vi "UI.vi"() -> ()   [LabVIEW 2016, in "动力环境.lvlib"]
uses:
  C:/Program Files (x86)/National Instruments/LabVIEW 2016/vi.lib/ActorFramework/Actor/Actor.lvclass
  DAM0200-Relay/DAM0200-Relay/DAM0200-Relay.lvclass
  EPEVER-MPPT/EPEVER-MPPT/EPEVER-MPPT.lvclass
  GPS/GPS/GPS.lvclass
  GPS/GPS/GPS.lvclass/GPS.ctl
  EPEVER-MPPT/EPEVER-MPPT/EPEVER-MPPT.lvclass/EPEVER-MPPT.ctl
  DAM0200-Relay/DAM0200-Relay/DAM0200-Relay.lvclass/DAM0200-Relay.ctl
  <vilib>/ActorFramework/Message Enqueuer/Message Enqueuer.lvclass/Message Enqueuer.ctl
  <vilib>/ActorFramework/Message Enqueuer/Enqueue.vi
  C:/Program Files (x86)/National Instruments/LabVIEW 2016/vi.lib/ActorFramework/Message/Message.lvclass
  <vilib>/ActorFramework/Stop Msg/Stop Msg.lvclass
  <vilib>/ActorFramework/Message Priority Queue/Priority Enqueue.vi
  <vilib>/ActorFramework/Actor/Actor.lvclass
  <vilib>/ptbypt/NI_PtbyPt.lvlib
  <vilib>/Utility/config.llb/NI_LVConfig.lvlib
panel:
  in  "仪器自动断电":T1={"开关"=enum."关闭", "偏置"=0, "间隔"=30} {"间隔" format="%02.0f"; "偏置" format="%02.0f"}
  out "通电时间":dbl format="%#.1f"
  out "偏移距离":dbl
  out "起始GPS":cluster{"GPS纬度":dbl[], "GPS经度":dbl[]} {"GPS经度" format="%#.6f °"; "GPS纬度" format="%#.6f °"}
  out "GPS轨迹图":cluster{"GPS纬度":dbl[], "GPS经度":dbl[]}[](graph)
  in  "仪器电源开关":bool
  in  "摄像头电源开关":bool
  out "仪器电源":bool
  out "摄像头电源":bool
  in  "GPS纬度":dbl format="%#.6f °"
  in  "GPS经度":dbl format="%#.6f °"
  in  "电压":dbl format="%#.2f V"
  in  "湿度":dbl format="%#.2f %%"
  in  "温度":dbl format="%#.2f ℃"
  # "开关："
  # "起始（分）："
  # "间隔（分）："
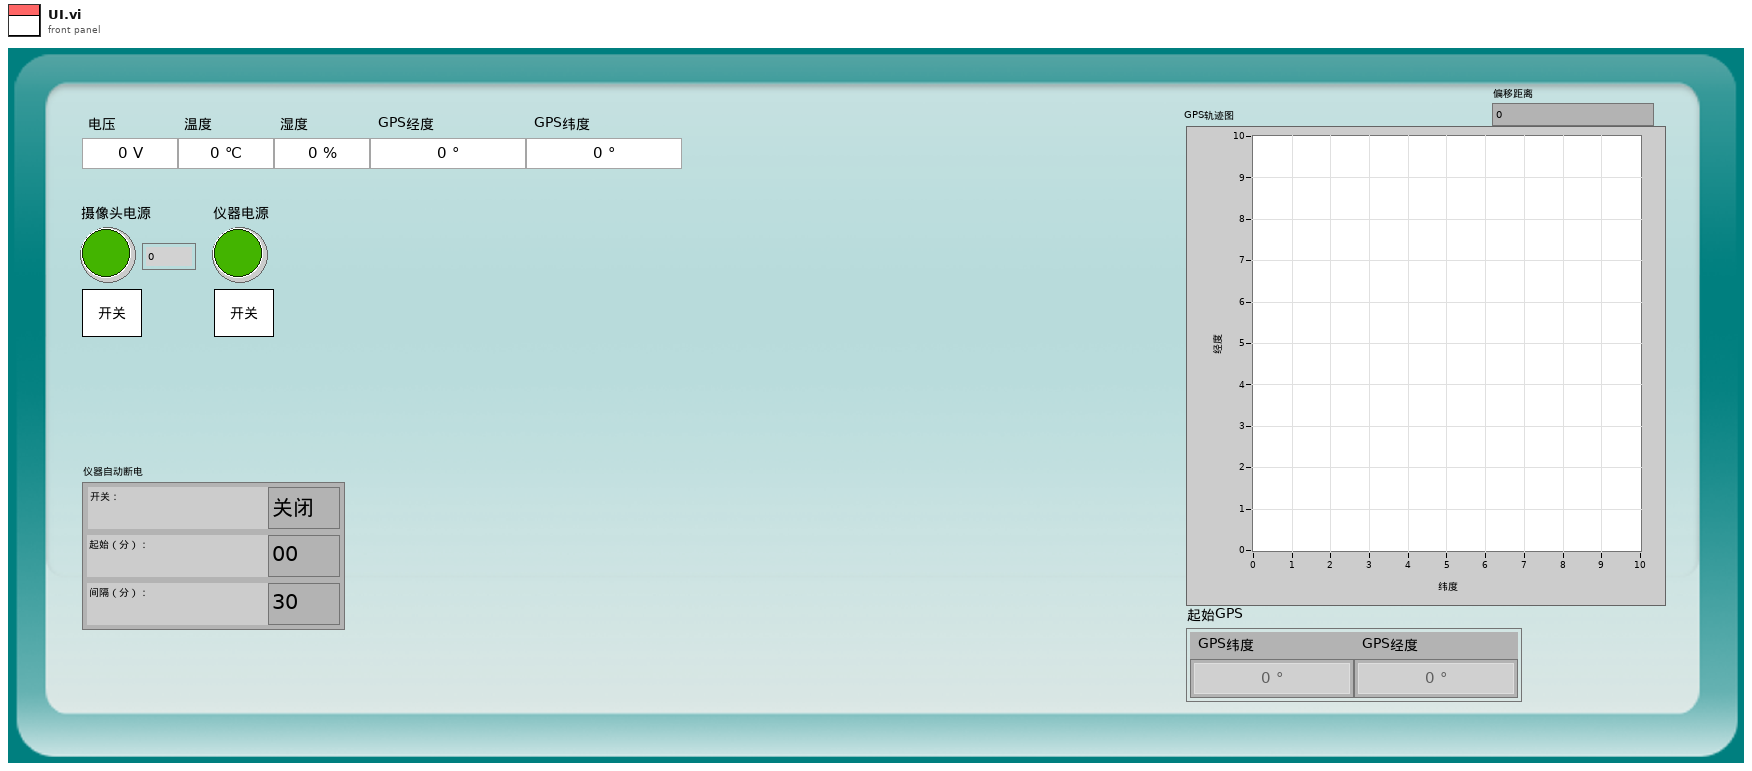
[diagram p1: front panel]
types:
  T1 = cluster{"开关":enum16{"关闭", "打开"}, "偏置":u16, "间隔":u16}
  T2 = cluster{"通电时间":timestamp, "通电超时？":bool, "低电压？":bool}
  T3 = typedef "报警信息字段定义.ctl" = cluster{"时间":timestamp, "参数":string, "元器件":string, "故障现象":string, "故障分析":string, "state":string, "code":string, "platform_alarm_code":string}
  T4 = typedef "NI_LVConfig.lvlib/Config Data RefNum.ctl" = refnum<k1>
  T5 = cluster{"时间":timestamp, "电压":dbl, "室温":dbl, "湿度":dbl, "GPS经度":dbl, "GPS纬度":dbl}
  T6 = typedef "LVDateTimeRec.ctl" = cluster{"秒数的小数部分":dbl, "秒":i32, "分":i32, "时":i32, "日":i32, "月":i32, "年":i32, "天数（周）":i32, "天数（年）":i32, "DST":i32}
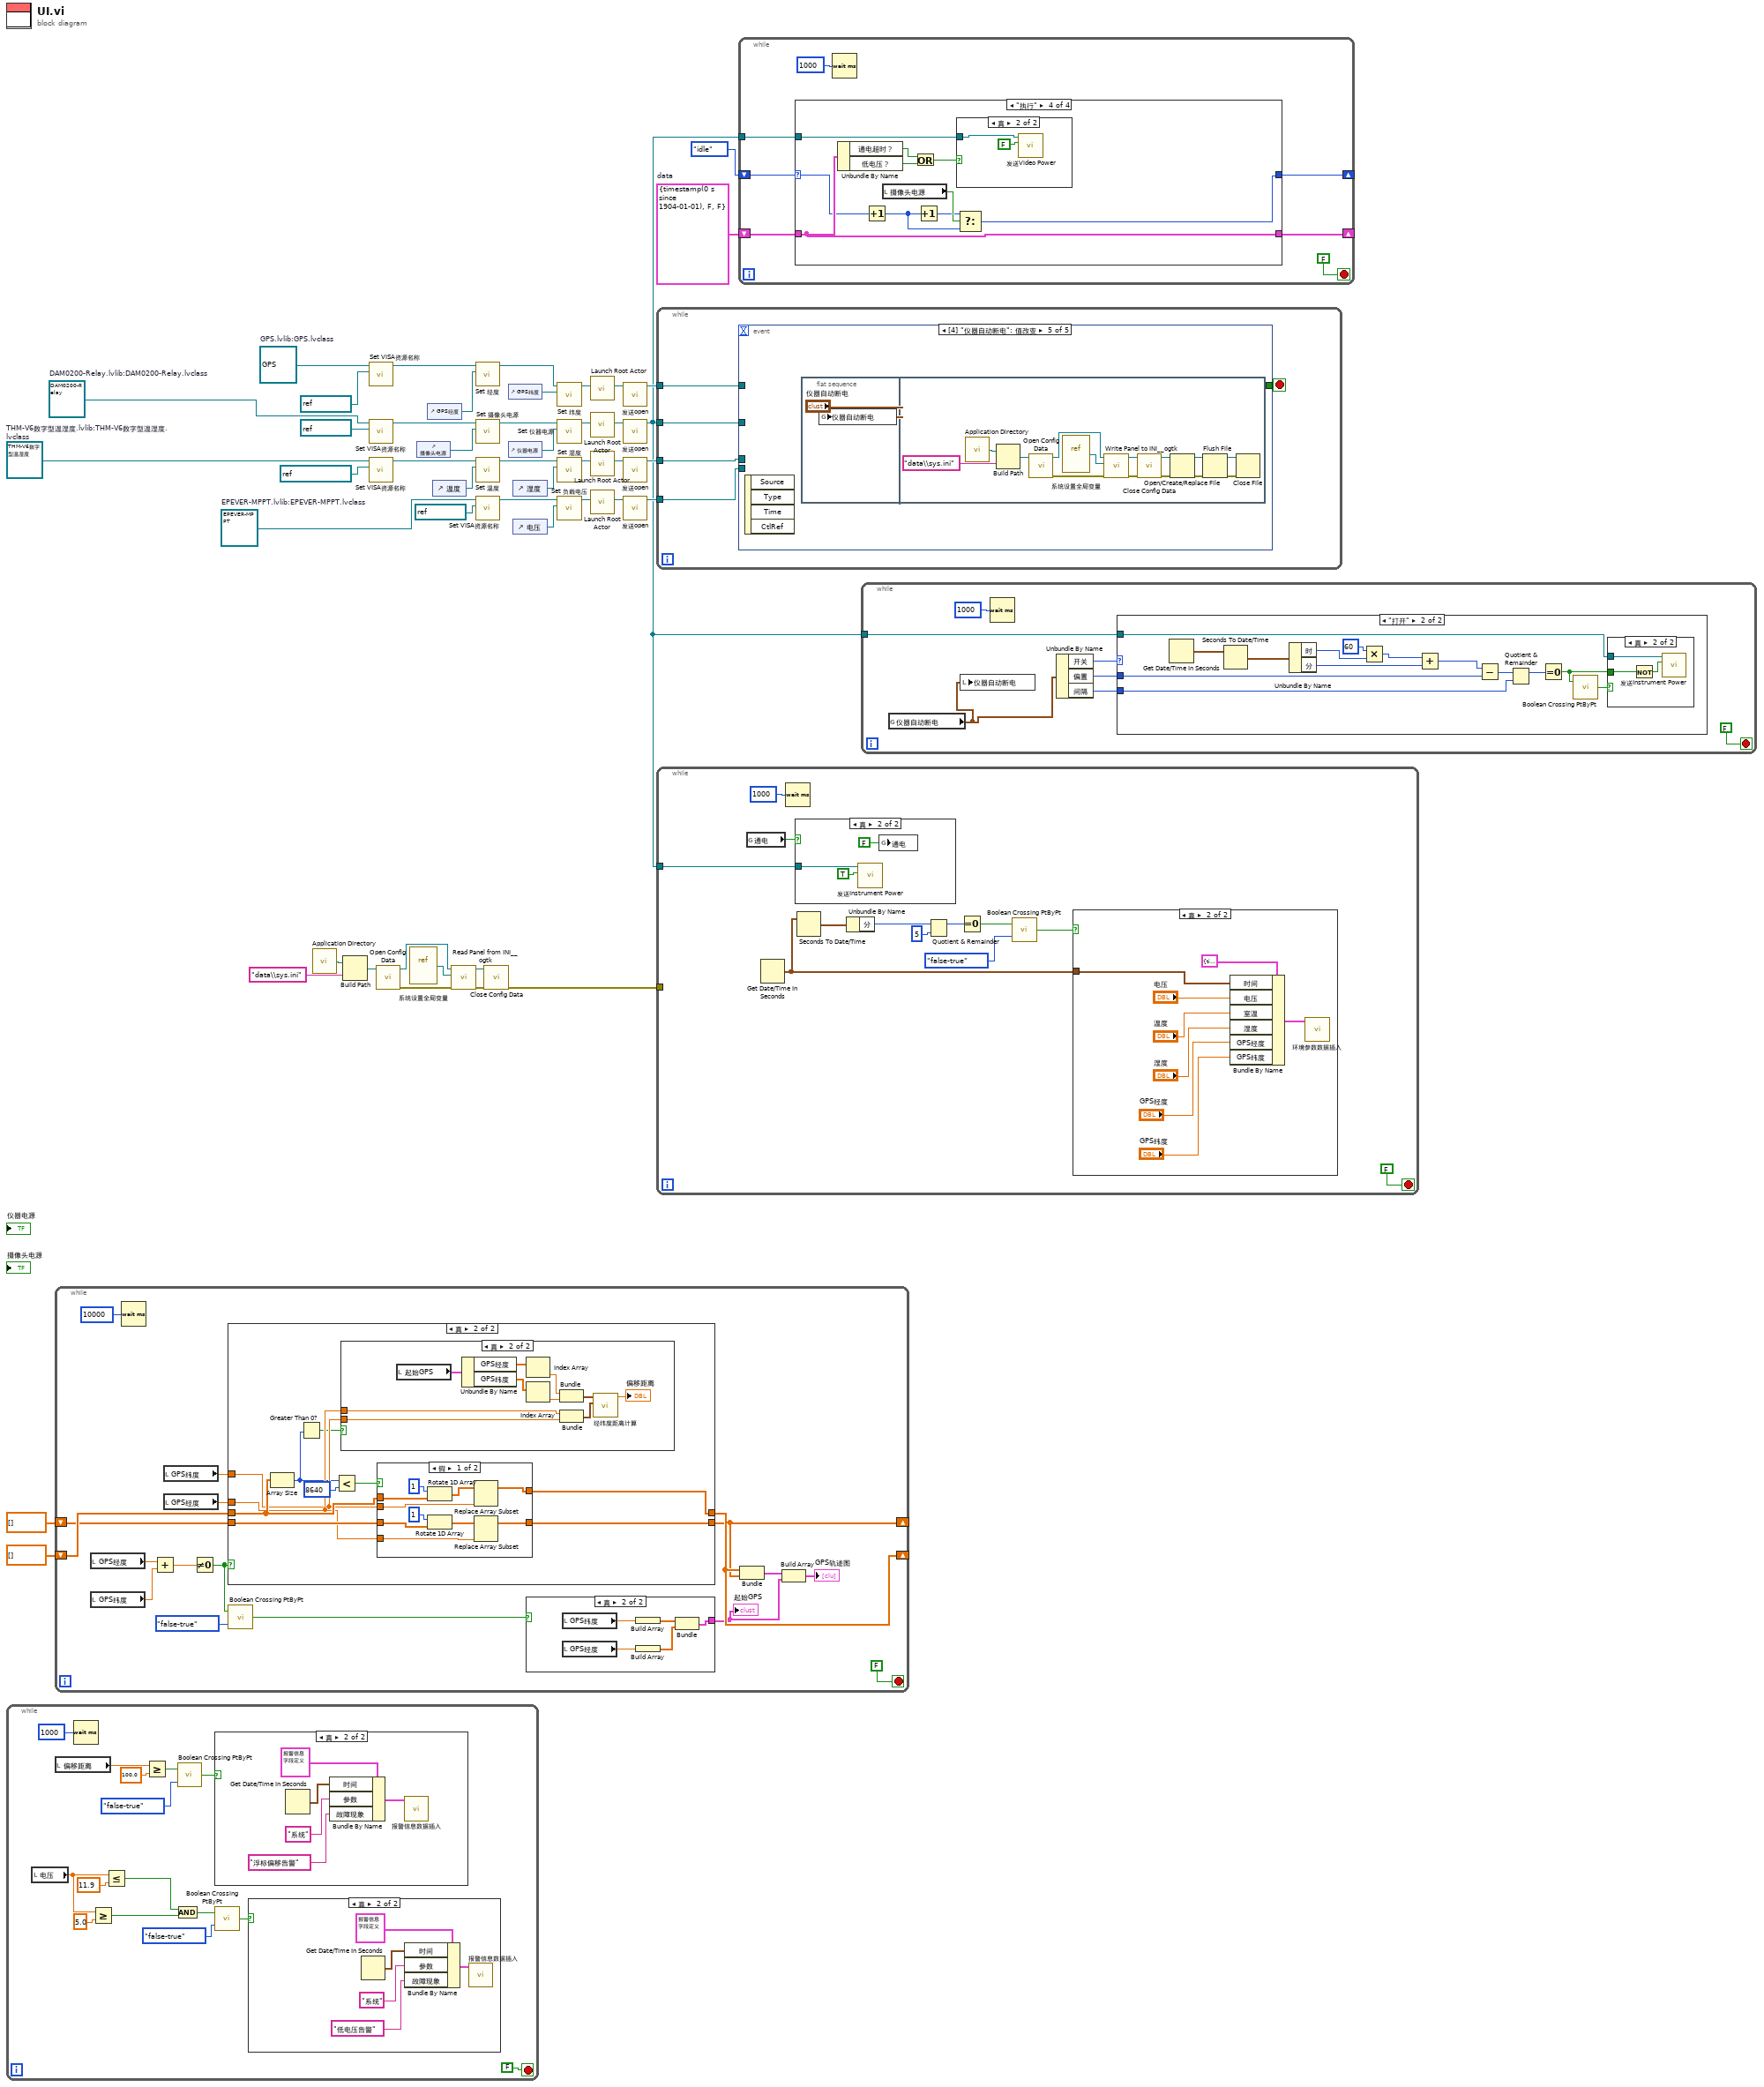
[diagram p0: block diagram]
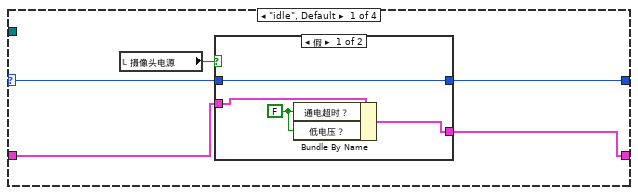
[diagram p4: hidden frame]
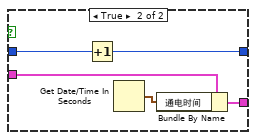
[diagram p5: hidden frame]
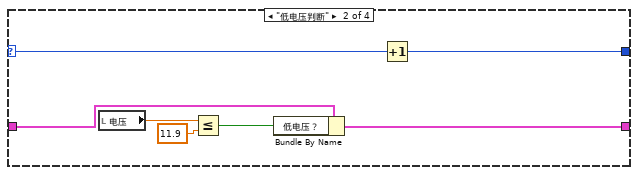
[diagram p6: hidden frame]
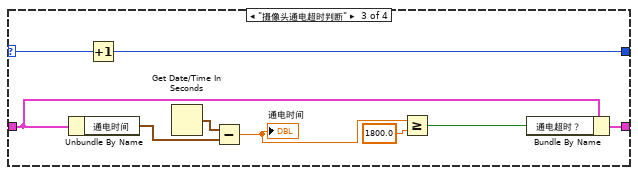
[diagram p7: hidden frame]
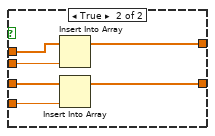
[diagram p13: hidden frame]
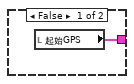
[diagram p14: hidden frame]
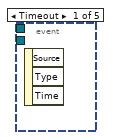
[diagram p17: hidden frame]
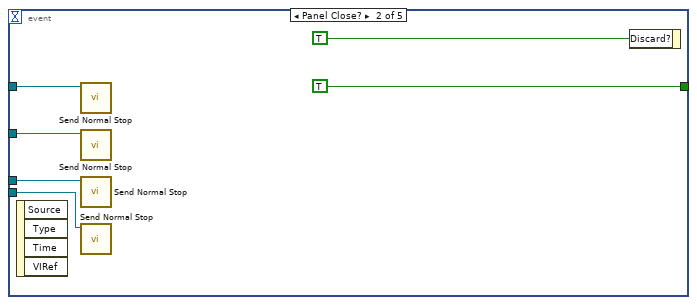
[diagram p18: hidden frame]
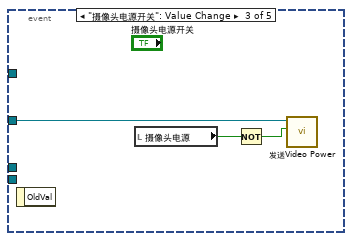
[diagram p19: hidden frame]
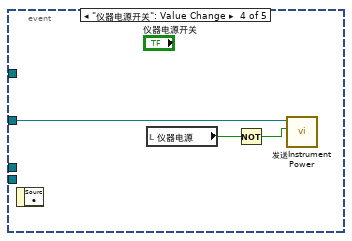
[diagram p20: hidden frame]
diagram:
  w11 = T2 {"通电时间"=timestamp(0 s since 1904-01-01), "通电超时？"=FALSE, "低电压？"=FALSE}  # data
  w23 = refnum<class "GPS.lvclass"> refnum  # GPS.lvlib:GPS.lvclass
  w31 = refnum<class "EPEVER-MPPT.lvclass"> refnum  # EPEVER-MPPT.lvlib:EPEVER-MPPT.lvclass
  w39 = refnum<class "DAM0200-Relay.lvclass"> refnum  # DAM0200-Relay.lvlib:DAM0200-Relay.lvclass
  w45 = refnum<class "THM-V6数字型温湿度.lvclass"> refnum  # THM-V6数字型温湿度.lvlib:THM-V6数字型温湿度.lvclass
  n1 = while {
    stop <- FALSE stop-if-true
    n2 = local read "电压"() -> (w51:dbl)
    n3 = local read "偏移距离"() -> (w61:dbl)
    n4 = Wait (ms)(milliseconds to wait=u32 1000 ("等待时间（毫秒）")) -> ()  [unwired: 1 out]
    n5 = Greater Or Equal?(x=w51, y=5.0) -> (x >= y?=w48:bool)
    n6 = Less Or Equal?(x=w51, y=11.9) -> (x <= y?=w52:bool)
    n7 = Greater Or Equal?(x=w61, y=100.0) -> (x >= y?=w59:bool)
    n8 = And(x=w52, y=w48) -> (x .and. y?=w49:bool)
    n9 = call <vilib>:"Boolean Crossing PtByPt.vi"("direction"=enum16{"either", "false-true", "true-false"}."false-true", "input"=w59) -> ("crossing"=w58:bool)  [unwired: 1 in]
    n10 = case shown="真" w58 {
      frame False {
      }
      frame True {
        n11 = Get Date/Time In Seconds() -> (seconds since 1Jan1904=w69:timestamp)
        n12 = Bundle By Name(cluster=T3 {"时间"=timestamp(0 s since 1904-01-01), "参数"="", "元器件"="", "故障现象"="", "故障分析"="", "state"="", "code"="", "platform_alarm_code"=""} ("data"), "时间"=w69, "参数"="系统", "故障现象"="浮标偏移告警") -> (w72:T3)
        n13 = call "报警信息数据插入.vi"("data"=w72) -> ()  [unwired: 9 in, 1 out]
      }
    }
    n14 = call <vilib>:"Boolean Crossing PtByPt.vi"("direction"=enum16{"either", "false-true", "true-false"}."false-true", "input"=w49) -> ("crossing"=w54:bool)  [unwired: 1 in]
    n15 = case shown="真" w54 {
      frame False {
      }
      frame True {
        n16 = Get Date/Time In Seconds() -> (seconds since 1Jan1904=w66:timestamp)
        n17 = Bundle By Name(cluster=T3 {"时间"=timestamp(0 s since 1904-01-01), "参数"="", "元器件"="", "故障现象"="", "故障分析"="", "state"="", "code"="", "platform_alarm_code"=""} ("data"), "时间"=w66, "参数"="系统", "故障现象"="低电压告警") -> (w63:T3)
        n18 = call "报警信息数据插入.vi"("data"=w63) -> ()  [unwired: 9 in, 1 out]
      }
    }
  }
  n19 = while {
    shift-right: [w78] -> _
    shift-left: dbl[] [] ("数组") -> [w80]
    shift-right: [w77] -> _
    shift-left: dbl[] [] ("数组") -> [w79]
    stop <- FALSE stop-if-true
    n20 = local read "GPS经度"() -> (w88:dbl)
    n21 = local read "GPS纬度"() -> (w87:dbl)
    n22 = Wait (ms)(milliseconds to wait=u32 10000 ("等待时间（毫秒）")) -> ()  [unwired: 1 out]
    n23 = Add(x=w88, y=w87) -> (x+y=w86:dbl)
    n24 = local read "GPS纬度"() -> (w82:dbl)
    n25 = local read "GPS经度"() -> (w81:dbl)
    n26 = Not Equal To 0?(x=w86) -> (x != 0?=w83:bool)
    n27 = case shown="真" w83 {
      tunnel: w82 -> [_ w94]
      tunnel: w81 -> [_ w95]
      tunnel: w80 -> [w91 w98]
      tunnel: w79 -> [w90 w100]
      tunnel: [w91 w101] -> w78
      tunnel: [w90 w99] -> w77
      frame False {
      }
      frame True {
        n28 = Array Size(array=w98) -> (size(s)=w93:i32)
        n29 = Greater Than 0?(x=w93) -> (x > 0?=w92:bool)
        n30 = Less?(x=w93, y=8640) -> (x < y?=w96:bool)
        n31 = case shown="真" w92 {
          tunnel: w95 -> [_ w105]
          tunnel: w94 -> [_ w104]
          frame False {
          }
          frame True {
            n32 = local read "起始GPS"() -> (w111:cluster{"GPS纬度":dbl[], "GPS经度":dbl[]})
            n33 = Unbundle By Name(w111) -> ("GPS经度"=w110:dbl[], "GPS纬度"=w109:dbl[])
            n34 = Index Array(array=w110) -> (element=w108:dbl)  [unwired: 1 in]
            n35 = Index Array(array=w109) -> (element=w107:dbl)  [unwired: 1 in]
            n36 = Bundle("GPS经度"=w108, "GPS纬度"=w107) -> (w106:cluster{"GPS经度":dbl, "GPS纬度":dbl})  [unwired: 1 in]
            n37 = Bundle("GPS经度"=w105, "GPS纬度"=w104) -> (w103:cluster{"GPS经度":dbl, "GPS纬度":dbl})  [unwired: 1 in]
            n38 = call "经纬度距离计算.vi"("结束位置"=w103, "起始位置"=w106) -> ("距离"=→"偏移距离":dbl)  [unwired: 9 in]
          }
        }
        n39 = case shown="假" w96 {
          tunnel: w94 -> [w116 w127]
          tunnel: [w115 w126] -> w101
          tunnel: w100 -> [w118 w125]
          tunnel: w95 -> [w113 w124]
          tunnel: [w112 w123] -> w99
          tunnel: w98 -> [w121 w122]
          frame False {
            n40 = Rotate 1D Array(1:w121, 2:1 ("n")) -> (0:w117:dbl[])
            n41 = Rotate 1D Array(1:w118, 2:1 ("n")) -> (0:w114:dbl[])
            n42 = Replace Array Subset(array=w117, new element=w116) -> (w115:dbl[])  [unwired: 1 in]
            n43 = Replace Array Subset(array=w114, new element=w113) -> (w112:dbl[])  [unwired: 1 in]
          }
          frame True {
            n44 = Insert Into Array(array=w122, new element=w127) -> (w126:dbl[])  [unwired: 1 in]
            n45 = Insert Into Array(array=w125, new element=w124) -> (w123:dbl[])  [unwired: 1 in]
          }
        }
      }
    }
    n46 = call <vilib>:"Boolean Crossing PtByPt.vi"("direction"=enum16{"either", "false-true", "true-false"}."false-true", "input"=w83) -> ("crossing"=w85:bool)  [unwired: 1 in]
    n47 = case shown="真" w85 {
      tunnel: [w128 w132] -> w75
      frame False {
        n48 = local read "起始GPS"() -> (w128:cluster{"GPS纬度":dbl[], "GPS经度":dbl[]})
      }
      frame True {
        n49 = local read "GPS纬度"() -> (w129:dbl)
        n50 = local read "GPS经度"() -> (w133:dbl)
        n51 = Build Array(w129) -> (w131:dbl[])
        n52 = Build Array(w133) -> (w130:dbl[])
        n53 = Bundle(w131, w130) -> (w132:cluster{dbl[], dbl[]})  [unwired: 1 in]
      }
    }
    "起始GPS" <- w75
    n54 = Bundle("数组"=w78, "数组"=w77) -> (w76:cluster{"数组":dbl[], "数组":dbl[]})  [unwired: 1 in]
    n55 = Build Array(w76, w75) -> (→"GPS轨迹图":cluster{"GPS纬度":dbl[], "GPS经度":dbl[]}[])
  }
  n56 = call <vilib>:"Application Directory.vi"() -> ("Application Directory"=w2:path)
  n57 = Build Path(base path=w2, name or relative path="data\\sys.ini" ("名称或相对路径")) -> (appended path=w4:path)
  n58 = call "Set VISA资源名称.vi"("VISA资源名称"=refnum<visa-resource-name> "COM7", "GPS in"=w23) -> ("GPS out"=w22:refnum<class "GPS.lvclass">)  [unwired: 9 in]
  n59 = call "Set VISA资源名称.vi"("VISA资源名称"=refnum<visa-resource-name> "COM2", "DAM0200-Relay in"=w39) -> ("DAM0200-Relay out"=w38:refnum<class "DAM0200-Relay.lvclass">)  [unwired: 9 in]
  n60 = call "Set VISA资源名称.vi"("VISA资源名称"=refnum<visa-resource-name> "COM3", "THM-V6数字型温湿度 in"=w45) -> ("THM-V6数字型温湿度 out"=w46:refnum<class "THM-V6数字型温湿度.lvclass">)  [unwired: 9 in]
  n61 = call <vilib>:"Open Config Data.vi"("configuration file path"=w4) -> ("error out"=w8:errorcluster, "refnum"=w5:T4)  [unwired: 8 in, 1 out]
  n62 = vi-ref "系统设置全局变量.vi"() -> (w6:refnum<vi>)
  n63 = control-ref of="摄像头电源"() -> (w35:refnum<vi>)
  n64 = control-ref of="GPS经度"() -> (w16:refnum<vi>)
  n65 = control-ref of="温度"() -> (w43:refnum<vi>)
  n66 = call <userlib>:"Read Panel from INI__ogtk.vi"("error in (no error)"=w8, "VI ref"=w6, "refnum"=w5) -> ("error out"=w9:errorcluster, "refnum out"=w7:T4)  [unwired: 7 in]
  n67 = call "Set 经度.vi"("经度"=w16, "GPS in"=w22) -> ("GPS out"=w21:refnum<class "GPS.lvclass">)  [unwired: 9 in]
  n68 = call "Set 摄像头电源.vi"("摄像头电源"=w35, "DAM0200-Relay in"=w38) -> ("DAM0200-Relay out"=w37:refnum<class "DAM0200-Relay.lvclass">)  [unwired: 9 in]
  n69 = call "Set 温度.vi"("温度"=w43, "THM-V6数字型温湿度 in"=w46) -> ("THM-V6数字型温湿度 out"=w47:refnum<class "THM-V6数字型温湿度.lvclass">)  [unwired: 9 in]
  n70 = call "Set VISA资源名称.vi"("VISA资源名称"=refnum<visa-resource-name> "COM6", "EPEVER-MPPT in"=w31) -> ("EPEVER-MPPT out"=w30:refnum<class "EPEVER-MPPT.lvclass">)  [unwired: 9 in]
  n71 = call <vilib>:"Close Config Data.vi"("error in (no error)"=w9, "refnum"=w7) -> ("error out"=w1:errorcluster)  [unwired: 8 in, 1 out]
  n72 = control-ref of="GPS纬度"() -> (w15:refnum<vi>)
  n73 = control-ref of="仪器电源"() -> (w34:refnum<vi>)
  n74 = control-ref of="湿度"() -> (w42:refnum<vi>)
  n75 = control-ref of="电压"() -> (w28:refnum<vi>)
  n76 = call "Set 纬度.vi"("纬度"=w15, "GPS in"=w21) -> ("GPS out"=w20:refnum<class "GPS.lvclass">)  [unwired: 9 in]
  n77 = call "Set 仪器电源.vi"("仪器电源"=w34, "DAM0200-Relay in"=w37) -> ("DAM0200-Relay out"=w33:refnum<class "DAM0200-Relay.lvclass">)  [unwired: 9 in]
  n78 = call "Set 湿度.vi"("湿度"=w42, "THM-V6数字型温湿度 in"=w47) -> ("THM-V6数字型温湿度 out"=w24:refnum<class "THM-V6数字型温湿度.lvclass">)  [unwired: 9 in]
  n79 = call "Set 负载电压.vi"("负载电压"=w28, "EPEVER-MPPT in"=w30) -> ("EPEVER-MPPT out"=w27:refnum<class "EPEVER-MPPT.lvclass">)  [unwired: 9 in]
  n80 = call <vilib>:"Launch Root Actor.vi"("Actor"=w20) -> ("Actor's Enqueuer"=w19:refnum<class "Message Enqueuer.lvclass">)  [unwired: 9 in, 1 out]
  n81 = call <vilib>:"Launch Root Actor.vi"("Actor"=w33) -> ("Actor's Enqueuer"=w32:refnum<class "Message Enqueuer.lvclass">)  [unwired: 9 in, 1 out]
  n82 = call <vilib>:"Launch Root Actor.vi"("Actor"=w24) -> ("Actor's Enqueuer"=w41:refnum<class "Message Enqueuer.lvclass">)  [unwired: 9 in, 1 out]
  n83 = call <vilib>:"Launch Root Actor.vi"("Actor"=w27) -> ("Actor's Enqueuer"=w26:refnum<class "Message Enqueuer.lvclass">)  [unwired: 9 in, 1 out]
  n84 = call "发送open.vi"("Message Enqueuer"=w19) -> ("Message Enqueuer out"=w18:refnum<class "Message Enqueuer.lvclass">)  [unwired: 9 in, 1 out]
  n85 = call "发送open.vi"("Message Enqueuer"=w32) -> ("Message Enqueuer out"=w10:refnum<class "Message Enqueuer.lvclass">)  [unwired: 9 in, 1 out]
  n86 = call "发送open.vi"("Message Enqueuer"=w41) -> ("Message Enqueuer out"=w40:refnum<class "Message Enqueuer.lvclass">)  [unwired: 9 in, 1 out]
  n87 = call "发送open.vi"("Message Enqueuer"=w26) -> ("Message Enqueuer out"=w25:refnum<class "Message Enqueuer.lvclass">)  [unwired: 9 in, 1 out]
  n88 = while {
    tunnel: w40 -> [w137]
    tunnel: w10 -> [w136]
    tunnel: w25 -> [w135]
    tunnel: w18 -> [w134]
    stop <- w138 stop-if-true
    n89 = event shown="[4] \"仪器自动断电\": 值改变" {
      selector: _ -> [_ _ _ _ _]
      dyn-events: _ -> [_ _ _ _ _]
      timeout: _ -> [_ _ _ _ _]
      tunnel: [_ TRUE _ _ _] -> w138
      tunnel: w137 -> [_ w142 _ _ _]
      tunnel: w136 -> [_ w141 w147 w150 _]
      tunnel: w135 -> [_ w140 _ _ _]
      tunnel: w134 -> [_ w139 _ _ _]
      event Timeout {
        n90 = event-data() -> ()  [unwired: 1 in, 3 out]
      }
      event Panel Close? {
        n91 = event-data() -> ()  [unwired: 1 in, 4 out]
        n92 = call <vilib>:"Send Normal Stop.vi"("Message Enqueuer"=w139) -> ()  [unwired: 10 in, 1 out]
        n93 = call <vilib>:"Send Normal Stop.vi"("Message Enqueuer"=w141) -> ()  [unwired: 10 in, 1 out]
        n94 = call <vilib>:"Send Normal Stop.vi"("Message Enqueuer"=w142) -> ()  [unwired: 10 in, 1 out]
        n95 = call <vilib>:"Send Normal Stop.vi"("Message Enqueuer"=w140) -> ()  [unwired: 10 in, 1 out]
        n96 = event-data("Discard?"=TRUE ("放弃？")) -> ()  [unwired: 1 in, 1 out]
      }
      event "摄像头电源开关": Value Change {
        n97 = event-data() -> ()  [unwired: 1 in, 1 out]
        n98 = local read "摄像头电源"() -> (w146:bool)
        n99 = Not(x=w146) -> (.not. x?=w145:bool)
        n100 = call "发送Video Power.vi"("布尔"=w145, "Message Enqueuer"=w147) -> ()  [unwired: 8 in, 2 out]
      }
      event "仪器电源开关": Value Change {
        n101 = event-data() -> ()  [unwired: 1 in, 1 out]
        n102 = local read "仪器电源"() -> (w149:bool)
        n103 = Not(x=w149) -> (.not. x?=w148:bool)
        n104 = call "发送Instrument Power.vi"("布尔"=w148, "Message Enqueuer"=w150) -> ()  [unwired: 8 in, 2 out]
      }
      event "仪器自动断电": Value Change {
        n105 = event-data() -> ()  [unwired: 1 in, 4 out]
        n106 = flat-sequence {
          frame #0 {
            n107 = global write "系统设置全局变量.vi" "仪器自动断电"("仪器自动断电") -> ()
          }
          frame #1 {
            n108 = call <vilib>:"Application Directory.vi"() -> ("Application Directory"=w152:path)
            n109 = Build Path(base path=w152, name or relative path="data\\sys.ini" ("名称或相对路径")) -> (appended path=w154:path)
            n110 = call <vilib>:"Open Config Data.vi"("configuration file path"=w154) -> ("error out"=w158:errorcluster, "refnum"=w155:T4)  [unwired: 8 in, 1 out]
            n111 = vi-ref "系统设置全局变量.vi"() -> (w156:refnum<vi>)
            n112 = call <userlib>:"Write Panel to INI__ogtk.vi"("error in (no error)"=w158, "VI ref"=w156, "refnum"=w155) -> ("error out"=w159:errorcluster, "refnum out"=w157:T4)  [unwired: 7 in]
            n113 = call <vilib>:"Close Config Data.vi"("error in (no error)"=w159, "refnum"=w157) -> ("error out"=w164:errorcluster, "file path"=w165:path)  [unwired: 8 in]
            n114 = Open/Create/Replace File(file path (use dialog)=w165, error in=w164) -> (refnum out=w161:refnum<file>, error out=w160:errorcluster)  [unwired: 4 in, 1 out]
            n115 = Flush File(refnum=w161, error in=w160) -> (refnum out=w162:refnum<file>, error out=w163:errorcluster)
            n116 = Close File(refnum=w162, error in=w163) -> ()  [unwired: 2 out]
          }
        }
      }
    }
  }
  n117 = while {
    tunnel: w10 -> [w166]
    tunnel: w1 -> [_]
    stop <- FALSE stop-if-true
    n118 = global read "系统设置全局变量.vi" "通电"() -> (w167:bool)
    n119 = Get Date/Time In Seconds() -> (seconds since 1Jan1904=w175:timestamp)
    n120 = Wait (ms)(milliseconds to wait=u32 1000 ("等待时间（毫秒）")) -> ()  [unwired: 1 out]
    n121 = case shown="真" w167 {
      tunnel: w166 -> [_ w180]
      frame False {
      }
      frame True {
        n122 = call "发送Instrument Power.vi"("布尔"=TRUE, "Message Enqueuer"=w180) -> ()  [unwired: 8 in, 2 out]
        n123 = global write "系统设置全局变量.vi" "通电"(FALSE ("通电")) -> ()
      }
    }
    n124 = Seconds To Date/Time(time stamp (now)=w175) -> (date time rec=w176:T6)  [unwired: 1 in]
    n125 = Unbundle By Name(w176) -> ("分"=w174:i32)
    n126 = Quotient & Remainder(x=w174, y=5) -> (x-y*floor(x/y)=w172:i32)  [unwired: 1 out]
    n127 = Equal To 0?(x=w172) -> (x = 0?=w171:bool)
    n128 = call <vilib>:"Boolean Crossing PtByPt.vi"("direction"=enum16{"either", "false-true", "true-false"}."false-true", "input"=w171) -> ("crossing"=w169:bool)  [unwired: 1 in]
    n129 = case shown="真" w169 {
      tunnel: w175 -> [_ w181]
      frame False {
      }
      frame True {
        n130 = Bundle By Name(cluster=T5 {"时间"=timestamp(0 s since 1904-01-01), "电压"=0.0, "室温"=0.0, "湿度"=0.0, "GPS经度"=0.0, "GPS纬度"=0.0} ("data"), "时间"=w181, "电压"="电压", "室温"="温度", "湿度"="湿度", "GPS经度"="GPS经度", "GPS纬度"="GPS纬度") -> (w187:T5)
        n131 = call "环境参数数据插入.vi"("data"=w187) -> ()  [unwired: 9 in, 1 out]
      }
    }
  }
  n132 = while {
    shift-right: [w190] -> _
    shift-left: enum16{"idle", "低电压判断", "摄像头通电超时判断", "执行"}."idle" ("枚举") -> [w194]
    shift-right: [w191] -> _
    shift-left: w11 -> [w193]
    tunnel: w10 -> [w192]
    stop <- FALSE stop-if-true
    n133 = case shown="\"执行\"" w194 {
      selector: w194 -> [w197 w211 w221 w229]
      tunnel: w193 -> [w200 w216 w219 w235]
      tunnel: w192 -> [_ _ _ w231]
      tunnel: [w198 w215 w218 w235] -> w191
      tunnel: [w196 w210 w220 w226] -> w190
      frame "idle", Default {
        n134 = local read "摄像头电源"() -> (w199:bool)
        n135 = case shown="假" w199 {
          tunnel: w200 -> [w204 w209]
          tunnel: [w203 w208] -> w198
          tunnel: w197 -> [w201 w206]
          tunnel: [w201 w205] -> w196
          frame False {
            w202 = FALSE ("通电超时？")
            n136 = Bundle By Name(cluster=w204, "通电超时？"=w202, "低电压？"=w202) -> (w203:T2)
          }
          frame True {
            n137 = Increment(x=w206) -> (x+1=w205:enum16{"idle", "低电压判断", "摄像头通电超时判断", "执行"})
            n138 = Get Date/Time In Seconds() -> (seconds since 1Jan1904=w207:timestamp)
            n139 = Bundle By Name(cluster=w209, "通电时间"=w207) -> (w208:T2)
          }
        }
      }
      frame "低电压判断" {
        n140 = local read "电压"() -> (w214:dbl)
        n141 = Less Or Equal?(x=w214, y=11.9) -> (x <= y?=w213:bool)
        n142 = Bundle By Name(cluster=w216, "低电压？"=w213) -> (w215:T2)
        n143 = Increment(x=w211) -> (x+1=w210:enum16{"idle", "低电压判断", "摄像头通电超时判断", "执行"})
      }
      frame "摄像头通电超时判断" {
        n144 = Unbundle By Name(w219) -> ("通电时间"=w224:timestamp)
        n145 = Increment(x=w221) -> (x+1=w220:enum16{"idle", "低电压判断", "摄像头通电超时判断", "执行"})
        n146 = Get Date/Time In Seconds() -> (seconds since 1Jan1904=w225:timestamp)
        n147 = Subtract(x=w225, y=w224) -> (x-y=w223:dbl)
        "通电时间" <- w223
        n148 = Greater Or Equal?(x=w223, y=1800.0) -> (x >= y?=w217:bool)
        n149 = Bundle By Name(cluster=w219, "通电超时？"=w217) -> (w218:T2)
      }
      frame "执行" {
        n150 = Unbundle By Name(w235) -> ("通电超时？"=w233:bool, "低电压？"=w234:bool)
        n151 = Increment(x=w229) -> (x+1=w227:enum16{"idle", "低电压判断", "摄像头通电超时判断", "执行"})
        n152 = local read "摄像头电源"() -> (w230:bool)
        n153 = Or(x=w233, y=w234) -> (x .or. y?=w232:bool)
        n154 = Increment(x=w227) -> (x+1=w228:enum16{"idle", "低电压判断", "摄像头通电超时判断", "执行"})
        n155 = case shown="真" w232 {
          tunnel: w231 -> [_ w237]
          frame False {
          }
          frame True {
            n156 = call "发送Video Power.vi"("布尔"=FALSE, "Message Enqueuer"=w237) -> ()  [unwired: 8 in, 2 out]
          }
        }
        n157 = Select(t=w228, s=w230, f=w227) -> (s? t:f=w226:enum16{"idle", "低电压判断", "摄像头通电超时判断", "执行"})
      }
    }
    n158 = Wait (ms)(milliseconds to wait=u32 1000 ("等待时间（毫秒）")) -> ()  [unwired: 1 out]
  }
  n159 = while {
    tunnel: w10 -> [w239]
    stop <- FALSE stop-if-true
    n160 = global read "系统设置全局变量.vi" "仪器自动断电"() -> (w238:T1)
    n161 = local write "仪器自动断电"(w238) -> ()
    n162 = Wait (ms)(milliseconds to wait=u32 1000 ("等待时间（毫秒）")) -> ()  [unwired: 1 out]
    n163 = Unbundle By Name(w238) -> ("开关"=w242:enum16{"关闭", "打开"}, "偏置"=w241:u16, "间隔"=w240:u16)
    n164 = case shown="\"打开\"" w242 {
      tunnel: w241 -> [_ w254]
      tunnel: w240 -> [_ w250]
      tunnel: w239 -> [_ w255]
      frame "关闭", Default {
      }
      frame "打开" {
        n165 = Get Date/Time In Seconds() -> (seconds since 1Jan1904=w258:timestamp)
        n166 = Seconds To Date/Time(time stamp (now)=w258) -> (date time rec=w257:T6)  [unwired: 1 in]
        n167 = Unbundle By Name(w257) -> ("时"=w253:i32, "分"=w248:i32)
        n168 = Multiply(x=60, y=w253) -> (x*y=w251:i32)
        n169 = Add(x=w251, y=w248) -> (x+y=w247:i32)
        n170 = Subtract(x=w247, y=w254) -> (x-y=w246:i32)
        n171 = Quotient & Remainder(x=w246, y=w250) -> (x-y*floor(x/y)=w249:i32)  [unwired: 1 out]
        n172 = Equal To 0?(x=w249) -> (x = 0?=w245:bool)
        n173 = call <vilib>:"Boolean Crossing PtByPt.vi"("input"=w245) -> ("crossing"=w256:bool)  [unwired: 2 in]
        n174 = case shown="真" w256 {
          tunnel: w255 -> [_ w260]
          tunnel: w245 -> [_ w259]
          frame False {
          }
          frame True {
            n175 = Not(x=w259) -> (.not. x?=w261:bool)
            n176 = call "发送Instrument Power.vi"("布尔"=w261, "Message Enqueuer"=w260) -> ()  [unwired: 8 in, 2 out]
          }
        }
      }
    }
  }
